vi "wf2str.vi"(5 "fields":enum16{"microsecs", "freq", "max_v", "y"}[](array[ring]), 6 "Signal":waveform(i16), 7 "PrevTime":timestamp) -> (0 "error out":errorcluster, 2 "Table":string[][](table), 3 "NextTime":timestamp)   [LabVIEW 2010]
panel:
  out "concatenated string":string
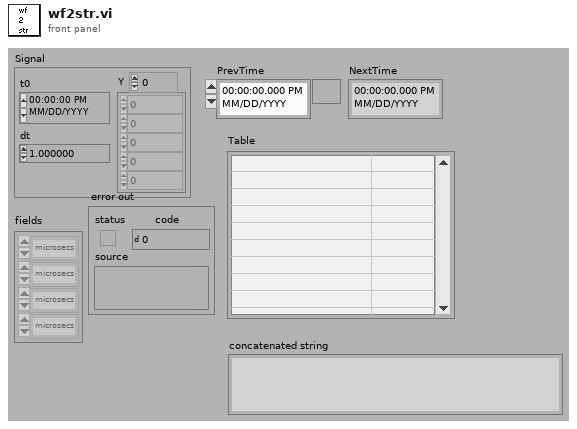
[diagram p1: front panel]
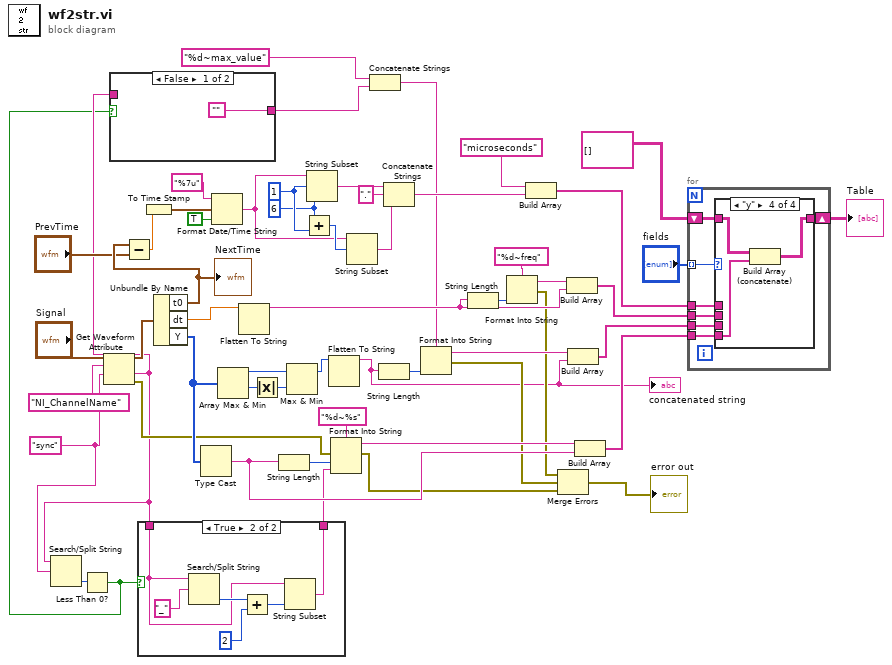
[diagram p0: block diagram]
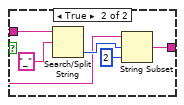
[diagram p2: hidden frame]
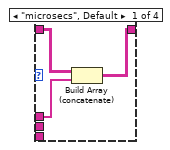
[diagram p4: hidden frame]
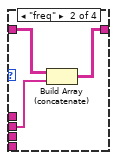
[diagram p5: hidden frame]
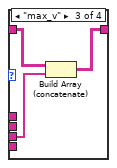
[diagram p6: hidden frame]
diagram:
  w3 = "sync" ("name")
  w38 = 6 ("length (rest)")
  w39 = 1 ("offset (0)")
  n1 = Get Waveform Attribute(5:w3, 6:"NI_ChannelName" ("name"), 7:"Signal") -> (0:w26:errorcluster, 1:w4:string, 3:w28:waveform(i16))  [unwired: 1 in, 1 out]
  n2 = Search/Split String(string=w4, search string/char (-)=w3) -> (offset of match=w2:i32)  [unwired: 1 in, 2 out]
  n3 = Less Than 0?(x=w2) -> (x < 0?=w1:bool)
  n4 = case shown="False" w1 {
    tunnel: ["" w58] -> w6
    tunnel: w4 -> [_ w57]
    frame False {
    }
    frame True {
      n5 = Search/Split String(string=w57, search string/char (-)="_" ("regular expression")) -> (offset of match=w59:i32)  [unwired: 1 in, 2 out]
      n6 = String Subset(string=w57, offset (0)=w59, length (rest)=2 ("length (rest)")) -> (substring=w58:string)
    }
  }
  n7 = case shown="True" w1 {
    tunnel: [w62 w67] -> w5
    tunnel: w4 -> [w62 w63]
    frame False {
    }
    frame True {
      n8 = Search/Split String(string=w63, search string/char (-)="_" ("regular expression")) -> (offset of match=w66:i32)  [unwired: 1 in, 2 out]
      n9 = Add(x=w66, y=2 ("length (rest)")) -> (x+y=w65:i32)
      n10 = String Subset(string=w63, length (rest)=w65) -> (substring=w67:string)  [unwired: 1 in]
    }
  }
  n11 = Unbundle By Name(w28) -> ("t0"=w13:timestamp, "dt"=w41:dbl, "Y"=w42:i16[])
  "NextTime" <- w13
  n12 = Subtract(x=w13, y="PrevTime") -> (x-y=w10:dbl)
  n13 = To Time Stamp(1:w10) -> (0:w11:timestamp)
  n14 = Type Cast(x=w42) -> (*(type *) &x=w55:string)  [unwired: 1 in]
  n15 = Format Date/Time String(time format string (%c)="%7u", seconds (now)=w11, UTC format=TRUE) -> (date/time string=w34:string)
  n16 = Array Max & Min(array=w42) -> (max value=w31:i16, min value=w29:i16)  [unwired: 2 out]
  n17 = Flatten To String(anything=w41) -> (data string=w51:string)  [unwired: 3 in, 2 out]
  n18 = Absolute Value(x=w29) -> (abs(x)=w30:i16)
  n19 = String Length(string=w55) -> (length=w43:i32)
  n20 = Max & Min(x=w31, y=w30) -> (max(x,y)=w32:i16)  [unwired: 1 out]
  n21 = Add(x=w38, y=w39) -> (x+y=w40:i32)
  n22 = String Subset(string=w34, offset (0)=w39, length (rest)=w38) -> (substring=w35:string)
  n23 = Flatten To String(anything=w32) -> (data string=w7:string)  [unwired: 3 in, 2 out]
  "concatenated string" <- w7
  n24 = Format Into String(format string="%d~%s", error in=w26, w43, w5) -> (resulting string=w54:string, error out=w23:errorcluster)  [unwired: 1 in]
  n25 = String Subset(string=w34, offset (0)=w40) -> (substring=w36:string)  [unwired: 1 in]
  n26 = Concatenate Strings("%d~max_value", w6) -> (w15:string)
  n27 = String Length(string=w7) -> (length=w52:i32)
  n28 = Concatenate Strings(w35, "." ("string"), w36) -> (w47:string)
  n29 = Format Into String(format string=w15, w52) -> (resulting string=w53:string, error out=w24:errorcluster)  [unwired: 2 in]
  n30 = String Length(string=w51) -> (length=w48:i32)
  n31 = Format Into String(format string="%d~freq", w48) -> (resulting string=w50:string, error out=w25:errorcluster)  [unwired: 2 in]
  n32 = Build Array("microseconds", w47) -> (w20:string[])
  n33 = Merge Errors(w25, w24, w23) -> (→"error out":errorcluster)
  n34 = Build Array(w50, w51) -> (w19:string[])
  n35 = Build Array(w53, w7) -> (w8:string[])
  n36 = Build Array(w54, w55) -> (w18:string[])
  n37 = for {
    tunnel: "fields" -> [w75] mode=indexing
    shift-right: [w70] -> w17
    shift-left: string[][] [] -> [w69]
    tunnel: w20 -> [w74]
    tunnel: w19 -> [w73]
    tunnel: w8 -> [w72]
    tunnel: w18 -> [w71]
    n38 = case shown="\"y\"" w75 {
      tunnel: w74 -> [w78 _ _ _]
      tunnel: w73 -> [_ w79 _ _]
      tunnel: w72 -> [_ _ w84 _]
      tunnel: w71 -> [_ _ _ w87]
      tunnel: [w77 w81 w82 w85] -> w70
      tunnel: w69 -> [w76 w80 w83 w86]
      frame "microsecs", Default {
        n39 = Build Array (concatenate)(w76, w78) -> (w77:string[][])
      }
      frame "freq" {
        n40 = Build Array (concatenate)(w80, w79) -> (w81:string[][])
      }
      frame "max_v" {
        n41 = Build Array (concatenate)(w83, w84) -> (w82:string[][])
      }
      frame "y" {
        n42 = Build Array (concatenate)(w86, w87) -> (w85:string[][])
      }
    }
  }
  "Table" <- w17
